vi "Read Address Pointer.vi"(8 "INC?":bool, 9 "Load?":bool, 10 "Load Value":u16, 11 "rollover":u16) -> (3 "count":u16)   [LabVIEW 2012]
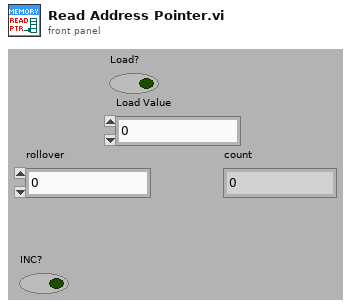
[diagram p1: front panel]
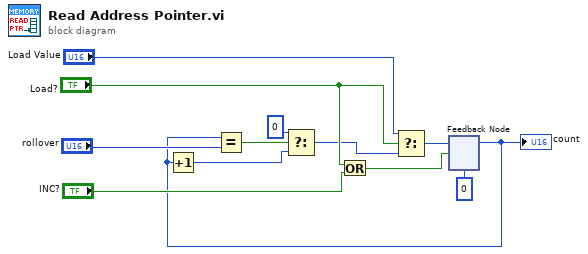
[diagram p0: block diagram]
diagram:
  n1 = Or(x="Load?", y="INC?") -> (x .or. y?=w2:bool)
  n2 = feedback #1(u16 0) -> (w1:u16)
  "count" <- w1
  n3 = Increment(x=w1) -> (x+1=w10:u16)
  n4 = Equal?(x=w1, y="rollover") -> (x = y?=w8:bool)
  n5 = Select(t=u16 0, s=w8, f=w10) -> (s? t:f=w4:u16)
  n6 = Select(t="Load Value", s="Load?", f=w4) -> (s? t:f=w3:u16)
  n7 = feedback-in #1(w3, w2) -> ()
